vi "RTDTemp.vi"() -> ()   [LabVIEW 2020]
uses:
  <vilib>/Analysis/baseanly.llb/Mean (DBL).vi
  Globals.vi
  <vilib>/Analysis/NI_AALBase.lvlib
panel:
  in  "stop (F)":bool
  out "Thermometer":dbl(slide) scale=0.0..200.0
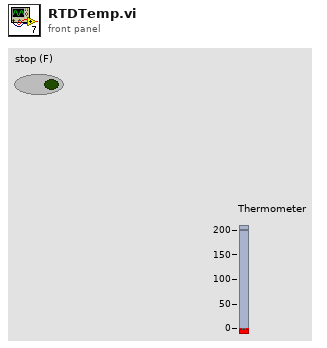
[diagram p1: front panel]
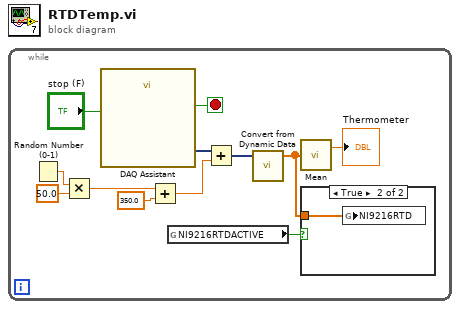
[diagram p0: block diagram]
diagram:
  n1 = while {
    stop <- w9 stop-if-true
    n2 = Random Number (0-1)() -> (number: 0 to 1=w6:dbl)
    n3 = Multiply(x=w6, y=50.0) -> (x*y=w3:dbl)
    n4 = call "DAQ Assistant"("stop (F)"="stop (F)") -> ("data"=w7:dynamicdata, "stopped"=w9:bool)  [unwired: 15 in, 2 out]
    n5 = Add(x=w3, y=350.0) -> (x+y=w1:dbl)
    n6 = global read "Globals.vi" "NI9216RTDACTIVE"() -> (w10:bool)
    n7 = Add(x=w7, y=w1) -> (x+y=w4:dynamicdata)
    n8 = call "Convert from Dynamic Data"("Dynamic Data Type"=w4) -> ("Array"=w11:dbl[])  [unwired: 3 in]
    n9 = call-poly <vilib>:"Mean.vi"("X"=w11) -> ("mean"=→"Thermometer":dbl)  [unwired: 1 out]
    n10 = case shown="True" w10 {
      tunnel: w11 -> [_ w13]
      frame False {
      }
      frame True {
        n11 = global write "Globals.vi" "NI9216RTD"(w13) -> ()
      }
    }
  }
